vi "clear 2552.vi"(1 "error in":errorcluster) -> (0 "error out":errorcluster)   [LabVIEW 2020]
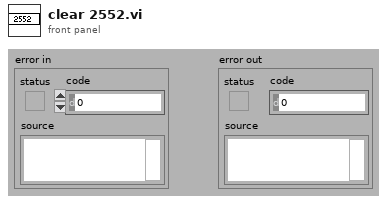
[diagram p1: front panel]
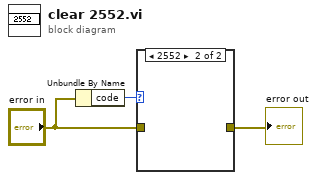
[diagram p0: block diagram]
diagram:
  n1 = Unbundle By Name("error in") -> ("code"=w3:i32)
  n2 = case shown="2552" w3 {
    tunnel: [w4 _] -> w1
    tunnel: "error in" -> [w4 _]
    frame 0, Default {
    }
    frame 2552 {
    }
  }
  "error out" <- w1
